vi "PH_Waveplate-GUI_6P.PC Overwrite Limits.vi"(0 "i ref in":refnum<vi>, 4 "Overwrite Limits?":bool, 5 "error in":errorcluster) -> (14 "i ref out":refnum<vi>, 19 "error out":errorcluster)   [LabVIEW 2014, in "PH_Waveplate-GUI_6P.lvlib"]
uses:
  PH_Waveplate-GUI_6P.lvlib
  PH_Waveplate-GUI_6P.Type.ctl
  PH_Basics/PH_Common/PH_Common.lvlib
  PH_Basics/PH_AxisGUI_BaseClass/PH_AxisGUI_BaseClass.lvlib
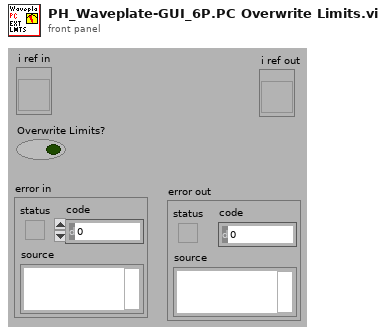
[diagram p1: front panel]
types:
  T1 = typedef "PH_Waveplate-GUI_6P.lvlib/PH_Waveplate-GUI_6P.Type.ctl" = u16
  T2 = typedef "PH_Waveplate-GUI_6P.lvlib/PH_Waveplate-GUI_6P.i attribute.ctl" = cluster{"GUI Refs":cluster{"Meter":refnum<vi>, "Extend Limits":refnum<vi>, "Type":refnum<vi>, "Target":refnum<vi>}, "Extend Waveplate Limit":bool, "Type":T1, "Limit":dbl}
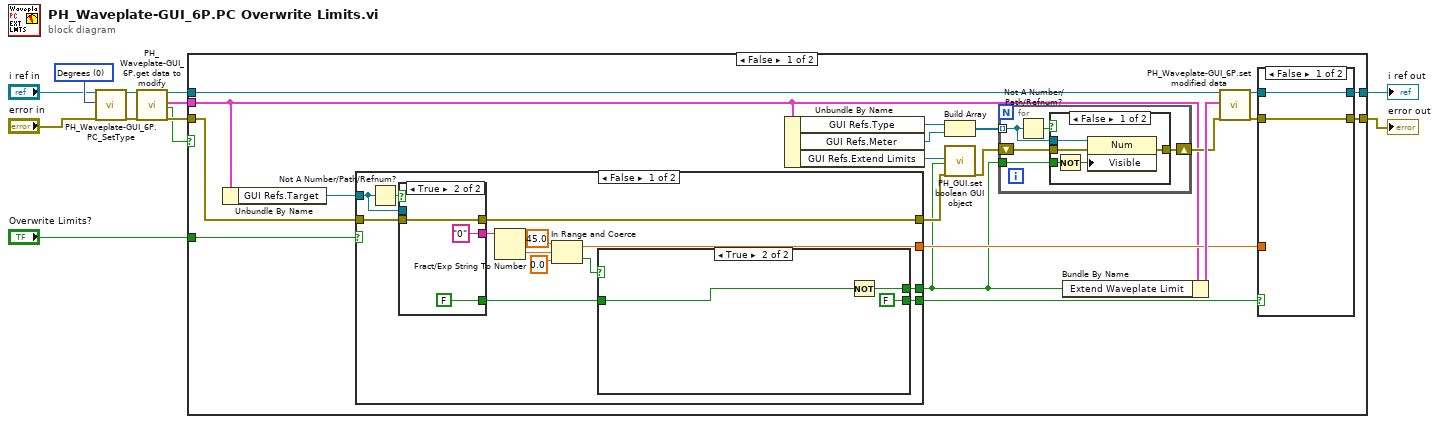
[diagram p0: block diagram]
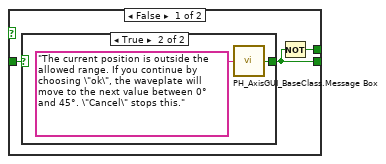
[diagram p3: hidden frame]
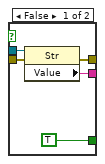
[diagram p5: hidden frame]
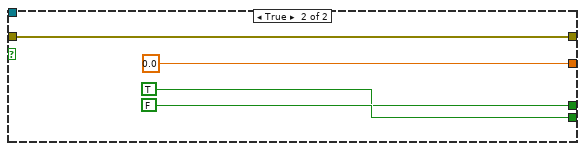
[diagram p6: hidden frame]
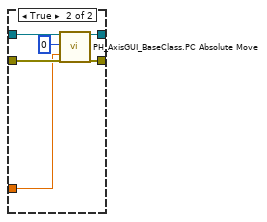
[diagram p7: hidden frame]
diagram:
  w5 = T1 0 items=["Degrees", "Percent"] ("Type")
  n1 = call "PH_Waveplate-GUI_6P.PC_SetType.vi"("VI in"="i ref in", "Type"=w5, "error in"="error in") -> ("VI out"=w4:refnum<vi>, "error out"=w3:errorcluster)  [unwired: 15 in]
  n2 = call "PH_Waveplate-GUI_6P.get data to modify.vi"("i ref in"=w4, "error in (no error)"=w3) -> ("i ref out"=w9:refnum<vi>, "i attribute"=w7:T2, "timed out"=w6:bool, "error out"=w8:errorcluster)  [unwired: 14 in]
  n3 = case shown="False" w6 {
    tunnel: "Overwrite Limits?" -> [w20 _]
    tunnel: [w26 w87] -> w11
    tunnel: [w24 w86] -> w10
    tunnel: w9 -> [w32 w87]
    tunnel: w8 -> [w23 w86]
    tunnel: w7 -> [w14 _]
    frame False {
      n4 = Unbundle By Name(w14) -> ("GUI Refs.Target"=w13:refnum<vi>)
      n5 = case shown="False" w20 {
        tunnel: w23 -> [w55 w76]
        tunnel: [w54 w76] -> w22
        tunnel: [w49 0.0 ("upper limit")] -> w21
        tunnel: [w47 FALSE] -> w18
        tunnel: [w45 TRUE] -> w19
        tunnel: w13 -> [w44 _]
        frame False {
          n6 = Not A Number/Path/Refnum?(number/path/refnum=w44) -> (NaN/Path/Refnum?=w56:bool)
          n7 = case shown="True" w56 {
            tunnel: w55 -> [w70 w73]
            tunnel: w44 -> [w69 _]
            tunnel: [w68 w73] -> w54
            tunnel: [w67 "0" ("Value")] -> w53
            tunnel: [TRUE FALSE] -> w48
            frame False {
              n8 = property class="Str"(reference=w69, error in=w70) -> (error out=w68:errorcluster, "Value"=w67:string)  [unwired: 1 out]
            }
            frame True {
            }
          }
          n9 = Fract/Exp String To Number(string=w53) -> (number=w52:dbl)  [unwired: 3 in, 1 out]
          n10 = In Range and Coerce(upper limit=45.0, x=w52, lower limit=0.0) -> (coerced(x)=w49:dbl, In Range?=w46:bool)
          n11 = case shown="True" w46 {
            tunnel: w48 -> [w59 w65]
            tunnel: [w57 FALSE ("OK?")] -> w47
            tunnel: [w58 w64] -> w45
            frame False {
              n12 = case shown="True" w59 {
                selector: w59 -> [w60 _]
                tunnel: [w60 w61] -> w57
                frame False {
                }
                frame True {
                  n13 = call "PH_AxisGUI_BaseClass.Message Box.vi"("String"="The current position is outside the allowed range. If you continue by choosing \"ok\", the waveplate will move to the next value between 0° and 45°. \"Cancel\" stops this.") -> ("OK?"=w61:bool)
                }
              }
              n14 = Not(x=w57) -> (.not. x?=w58:bool)
            }
            frame True {
              n15 = Not(x=w65) -> (.not. x?=w64:bool)
            }
          }
        }
        frame True {
        }
      }
      n16 = Unbundle By Name(w14) -> ("GUI Refs.Type"=w17:refnum<vi>, "GUI Refs.Meter"=w16:refnum<vi>, "GUI Refs.Extend Limits"=w30:refnum<vi>)
      n17 = Build Array(w17, w16) -> (w15:refnum<vi>[])
      n18 = call "PH_GUI.set boolean GUI object.vi"("Boolean Knob GUI Ref"=w30, "Value"=w19, "error in (no error)"=w22) -> ("error out"=w29:errorcluster)  [unwired: 16 in]
      n19 = for {
        tunnel: w19 -> [w34]
        tunnel: w15 -> [w33] mode=indexing
        shift-right: [w35] -> w28
        shift-left: w29 -> [w37]
        n20 = Not A Number/Path/Refnum?(number/path/refnum=w33) -> (NaN/Path/Refnum?=w36:bool)
        n21 = case shown="False" w36 {
          tunnel: w37 -> [w42 w43]
          tunnel: w33 -> [w41 _]
          tunnel: [w40 w43] -> w35
          tunnel: w34 -> [w39 _]
          frame False {
            n22 = Not(x=w39) -> (.not. x?=w38:bool)
            n23 = property class="Num"(reference=w41, error in=w42, "Visible"=w38) -> (error out=w40:errorcluster)  [unwired: 1 out]
          }
          frame True {
          }
        }
      }
      n24 = Bundle By Name(cluster=w14, "Extend Waveplate Limit"=w19) -> (w31:T2)
      n25 = call "PH_Waveplate-GUI_6P.set modified data.vi"("i ref in"=w32, "i attribute"=w31, "error in (no error)"=w28) -> ("i ref out"=w27:refnum<vi>, "error out"=w25:errorcluster)  [unwired: 15 in]
      n26 = case shown="False" w18 {
        tunnel: w27 -> [w79 w85]
        tunnel: [w79 w84] -> w26
        tunnel: w25 -> [w78 w83]
        tunnel: [w78 w82] -> w24
        tunnel: w21 -> [_ w81]
        frame False {
        }
        frame True {
          n27 = call "PH_AxisGUI_BaseClass.PC Absolute Move.vi"("i ref in"=w85, "Axis"=0, "Position [Units]"=w81, "error in"=w83) -> ("i ref out"=w84:refnum<vi>, "error out"=w82:errorcluster)  [unwired: 14 in]
        }
      }
    }
    frame True {
    }
  }
  "error out" <- w10
  "i ref out" <- w11
